vi "ts_M1M3SupportExpansionFPGA.vi"() -> ()   [LabVIEW 2018]
uses:
  <vilib>/rvi/Emulation/niFpgaGetClockAttributes.vi
  <vilib>/rvi/Emulation/niFpgaSctlEmulationGetInTimedLoop.vi
  <vilib>/rvi/Emulation/niFpgaEmulationReportErrorSimple.vi
  <vilib>/rvi/eio/common/nirviEmuTemplateMethod_errors.vi
  <vilib>/rvi/Emulation/niFpgaProcessEmulError.vi
  <vilib>/rvi/Emulation/niFpgaCriticalErrorInLSC.vi
  <vilib>/eio/EIONode/EIONode.xnode
panel:
  out "Slot2":u32 format="%032b"
  out "Slot1":sgl[](array[numeric]) format="%.3g"
  in  "Sample":bool
  # "Set Sample to TRUE then read Slot1 and Slot2"
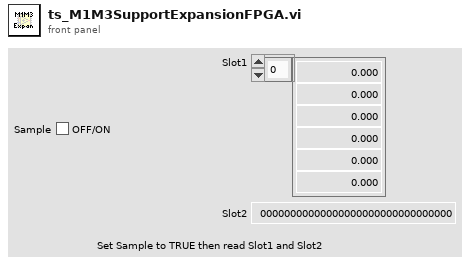
[diagram p1: front panel]
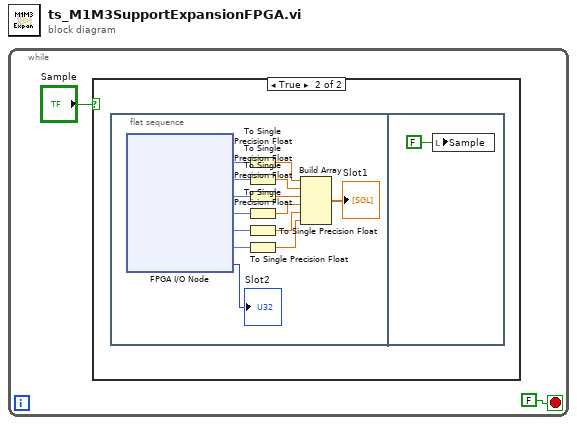
[diagram p0: block diagram]
diagram:
  n1 = while {
    stop <- FALSE stop-if-true
    n2 = case shown="True" "Sample" {
      frame False {
      }
      frame True {
        n3 = flat-sequence {
          frame #0 {
            n4 = xnode "FPGA I/O Node"() -> ("Slot1/AI0"=w16:fxp<+/-,24,5>, "Slot1/AI1"=w15:fxp<+/-,24,5>, "Slot1/AI2"=w14:fxp<+/-,24,5>, "Slot1/AI3"=w13:fxp<+/-,24,5>, "Slot1/AI4"=w12:fxp<+/-,24,5>, "Slot1/AI5"=w11:fxp<+/-,24,5>, "Slot2/DI31:0"=→"Slot2":u32)  [unwired: 7 in, 7 out]
            n5 = To Single Precision Float(number=w16) -> (single precision float=w10:sgl)
            n6 = To Single Precision Float(number=w15) -> (single precision float=w9:sgl)
            n7 = To Single Precision Float(number=w14) -> (single precision float=w8:sgl)
            n8 = To Single Precision Float(number=w13) -> (single precision float=w7:sgl)
            n9 = To Single Precision Float(number=w12) -> (single precision float=w6:sgl)
            n10 = To Single Precision Float(number=w11) -> (single precision float=w5:sgl)
            n11 = Build Array(w10, w9, w8, w7, w6, w5) -> (→"Slot1":sgl[])
          }
          frame #1 {
            n12 = local write "Sample"(FALSE ("Sample")) -> ()
          }
        }
      }
    }
  }
